vi "Convert String to Variant.vi"(8 "error in (no error)":errorcluster, 10 "Type String":string, 11 "Value String":string) -> (0 "error out":errorcluster, 2 "Variant":variant)   [LabVIEW 2018, in "Test.lvclass"]
doc: "Converts a string in the format \"Data Value//Data Type\" first to a string and data type enum, and then into a variant of the correct data type"
uses:
  Test.lvclass
  <vilib>/Utility/Data Type/Type Definitions/Data Type.ctl
  <vilib>/Utility/error.llb/Error Cluster From Error Code.vi
  <vilib>/ErrorRing/Error Ring.xnode
  <vilib>/Utility/Data Type/NI_Data Type.lvlib
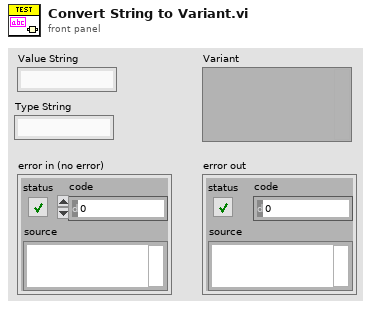
[diagram p1: front panel]
types:
  T1 = typedef "NI_Data Type.lvlib/Data Type.ctl" = enum8{"Invalid Type", "Void", "I8", "I16", "I32", "I64", "U8", "U16", "U32", "U64", "Single Float", "Double Float", "Extended Float", "Single Complex", "Double Complex", "Extended Complex", "Enum U8", "Enum U16", "Enum U32", "Enum U64", "Single Float With Unit", "Double Float With Unit", "Extended Float With Unit", "Single Complex with Unit", "Double Complex with Unit", "Extended Complex with Unit", "Boolean", "String", "Path", "Picture", "Tag", "Array", "Cluster", "Variant", "LV Variant", "Waveform", "Timestamp", "Digital Waveform", "Digital Data", "ExpressData", "Refnum", "External Data", "VI", "Poly VI", "LabVIEW Class Instance", "Fixed Point"}
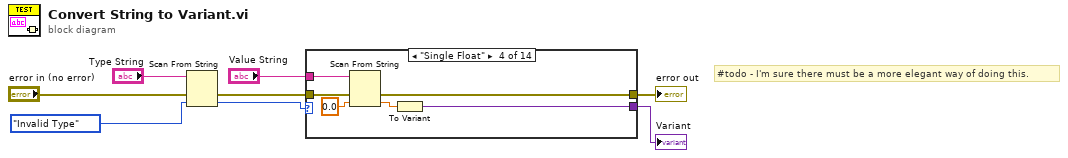
[diagram p0: block diagram]
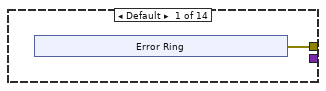
[diagram p2: hidden frame]
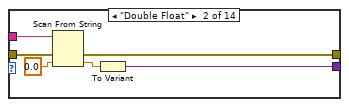
[diagram p3: hidden frame]
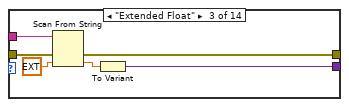
[diagram p4: hidden frame]
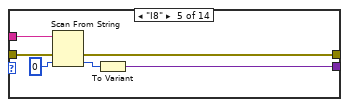
[diagram p5: hidden frame]
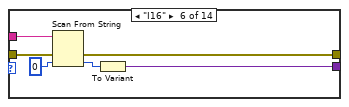
[diagram p6: hidden frame]
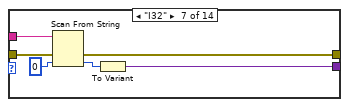
[diagram p7: hidden frame]
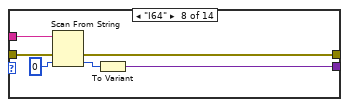
[diagram p8: hidden frame]
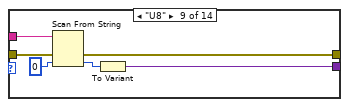
[diagram p9: hidden frame]
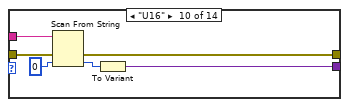
[diagram p10: hidden frame]
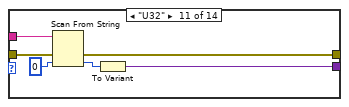
[diagram p11: hidden frame]
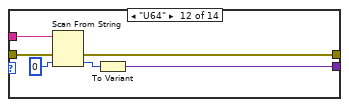
[diagram p12: hidden frame]
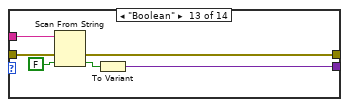
[diagram p13: hidden frame]
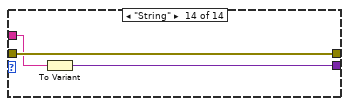
[diagram p14: hidden frame]
diagram:
  # "#todo - I'm sure there must be a more elegant way of doing this."
  n1 = Scan From String(input string="Type String", error in="error in (no error)", default 1=Data_Type."Invalid Type" ("Data Type")) -> (error out=w5:errorcluster, output 1=w3:T1)  [unwired: 2 in, 2 out]
  n2 = case shown="\"Single Float\"" w3 {
    tunnel: [_ w20 w26 w32 w38 w44 w50 w56 w62 w68 w74 w80 w86 w89] -> w8
    tunnel: [w9 w19 w25 w31 w37 w43 w49 w55 w61 w67 w73 w79 w85 w88] -> w7
    tunnel: w5 -> [_ w17 w23 w29 w35 w41 w47 w53 w59 w65 w71 w77 w83 w88]
    tunnel: "Value String" -> [_ w16 w22 w28 w34 w40 w46 w52 w58 w64 w70 w76 w82 w87]
    frame Default {
      n3 = xnode "Error Ring"() -> ("error out"=w9:errorcluster)
    }
    frame "Double Float" {
      n4 = Scan From String(input string=w16, error in=w17, default 1=0.0 ("default value 1")) -> (error out=w19:errorcluster, output 1=w18:dbl)  [unwired: 2 in, 2 out]
      n5 = To Variant(anything=w18) -> (Variant=w20:variant)
    }
    frame "Extended Float" {
      n6 = Scan From String(input string=w22, error in=w23, default 1=ext 0.0 ("default value 1")) -> (error out=w25:errorcluster, output 1=w24:ext)  [unwired: 2 in, 2 out]
      n7 = To Variant(anything=w24) -> (Variant=w26:variant)
    }
    frame "Single Float" {
      n8 = Scan From String(input string=w28, error in=w29, default 1=sgl 0.0 ("default value 1")) -> (error out=w31:errorcluster, output 1=w30:sgl)  [unwired: 2 in, 2 out]
      n9 = To Variant(anything=w30) -> (Variant=w32:variant)
    }
    frame "I8" {
      n10 = Scan From String(input string=w34, error in=w35, default 1=i8 0 ("default value 1")) -> (error out=w37:errorcluster, output 1=w36:i8)  [unwired: 2 in, 2 out]
      n11 = To Variant(anything=w36) -> (Variant=w38:variant)
    }
    frame "I16" {
      n12 = Scan From String(input string=w40, error in=w41, default 1=i16 0 ("default value 1")) -> (error out=w43:errorcluster, output 1=w42:i16)  [unwired: 2 in, 2 out]
      n13 = To Variant(anything=w42) -> (Variant=w44:variant)
    }
    frame "I32" {
      n14 = Scan From String(input string=w46, error in=w47, default 1=0 ("default value 1")) -> (error out=w49:errorcluster, output 1=w48:i32)  [unwired: 2 in, 2 out]
      n15 = To Variant(anything=w48) -> (Variant=w50:variant)
    }
    frame "I64" {
      n16 = Scan From String(input string=w52, error in=w53, default 1=i64 0 ("default value 1")) -> (error out=w55:errorcluster, output 1=w54:i64)  [unwired: 2 in, 2 out]
      n17 = To Variant(anything=w54) -> (Variant=w56:variant)
    }
    frame "U8" {
      n18 = Scan From String(input string=w58, error in=w59, default 1=u8 0 ("default value 1")) -> (error out=w61:errorcluster, output 1=w60:u8)  [unwired: 2 in, 2 out]
      n19 = To Variant(anything=w60) -> (Variant=w62:variant)
    }
    frame "U16" {
      n20 = Scan From String(input string=w64, error in=w65, default 1=u16 0 ("default value 1")) -> (error out=w67:errorcluster, output 1=w66:u16)  [unwired: 2 in, 2 out]
      n21 = To Variant(anything=w66) -> (Variant=w68:variant)
    }
    frame "U32" {
      n22 = Scan From String(input string=w70, error in=w71, default 1=u32 0 ("default value 1")) -> (error out=w73:errorcluster, output 1=w72:u32)  [unwired: 2 in, 2 out]
      n23 = To Variant(anything=w72) -> (Variant=w74:variant)
    }
    frame "U64" {
      n24 = Scan From String(input string=w76, error in=w77, default 1=u64 0 ("default value 1")) -> (error out=w79:errorcluster, output 1=w78:u64)  [unwired: 2 in, 2 out]
      n25 = To Variant(anything=w78) -> (Variant=w80:variant)
    }
    frame "Boolean" {
      n26 = Scan From String(input string=w82, error in=w83, default 1=FALSE) -> (error out=w85:errorcluster, output 1=w84:bool)  [unwired: 2 in, 2 out]
      n27 = To Variant(anything=w84) -> (Variant=w86:variant)
    }
    frame "String" {
      n28 = To Variant(anything=w87) -> (Variant=w89:variant)
    }
  }
  "Variant" <- w8
  "error out" <- w7
